vi "上传图片AOI.vi"(8 "error in (no error)":errorcluster caption="错误输入（无错误）", 10 "产品文件路径":string) -> (0 "error out":errorcluster, 1 "上传成功":bool)   [LabVIEW 2014]
uses:
  <vilib>/httpClient/MultipartData.ctl
  <vilib>/httpClient/LabVIEWHTTPClient.lvlib
panel:
  out "添加的路径":path
  out "ServerResponseBody_ANSI":string
  out "resulting string":string
  out "ServerResponseHead":string
  out "ServerResponseBody_UTF8":string
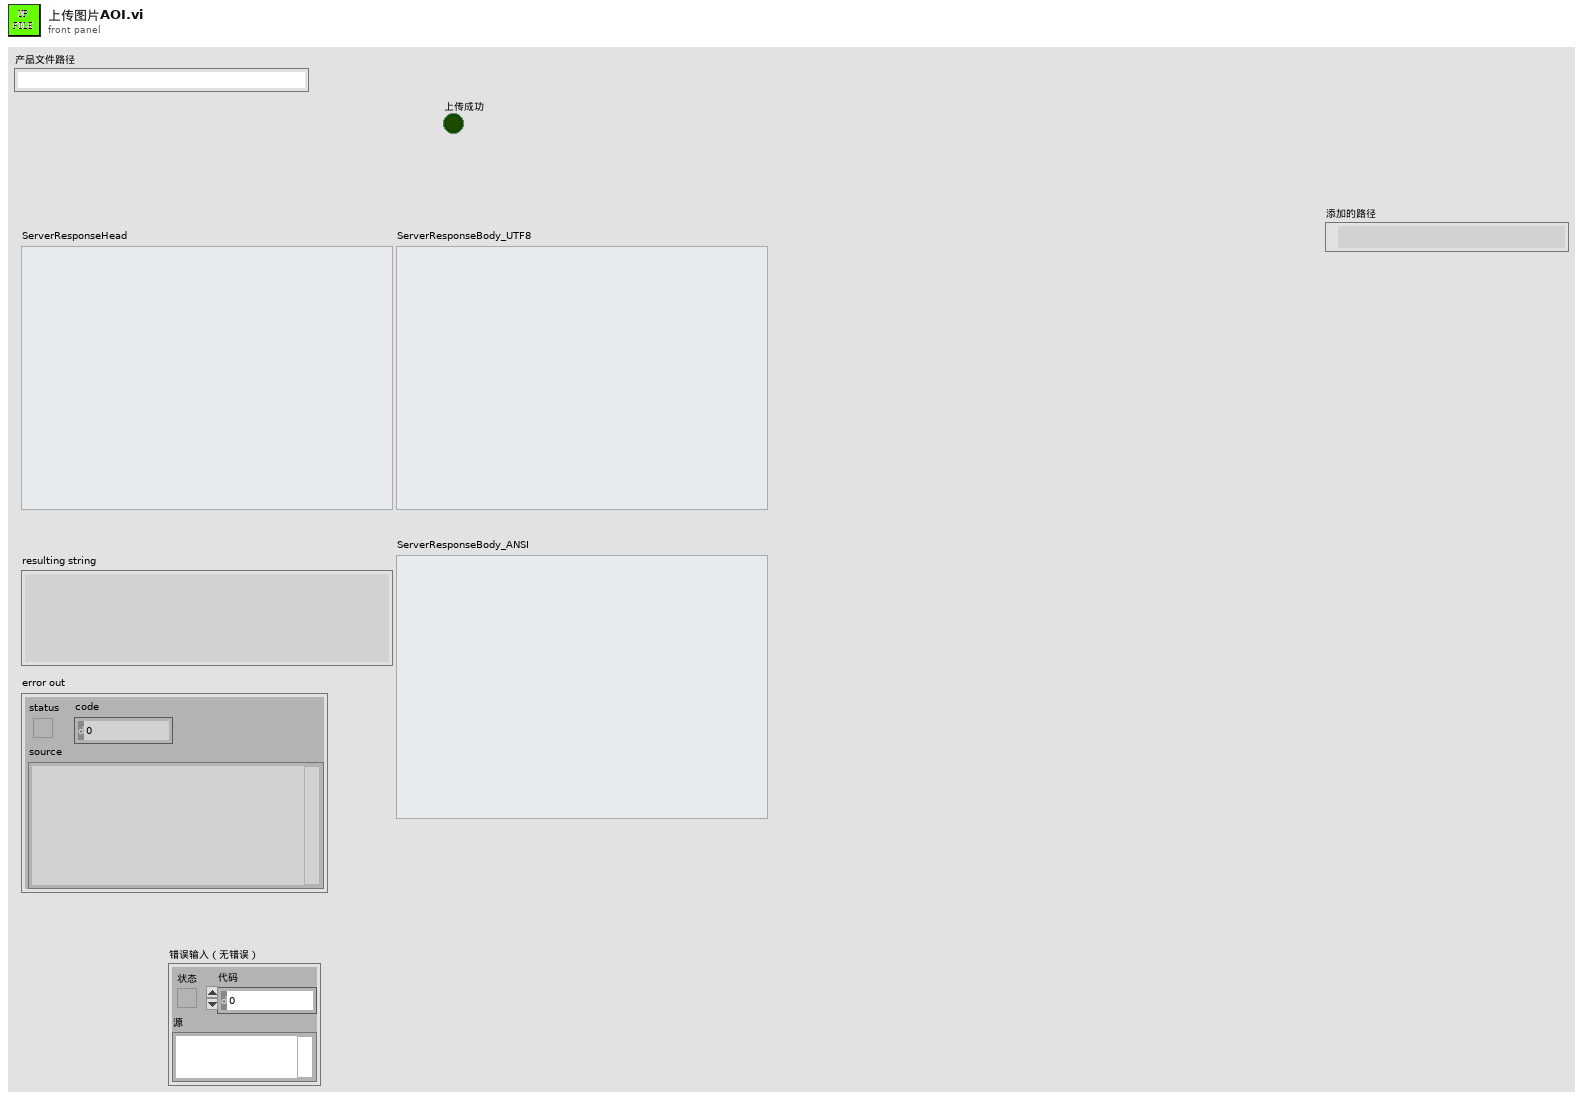
[diagram p1: front panel]
types:
  T1 = typedef "LabVIEWHTTPClient.lvlib/MultipartData.ctl" = cluster{"Name":string, "Value":string, "File":path, "Filename":string, "MIME type":string}
  T2 = typedef "LabVIEWHTTPClient.lvlib/ClientHandle.ctl" = refnum<k1>
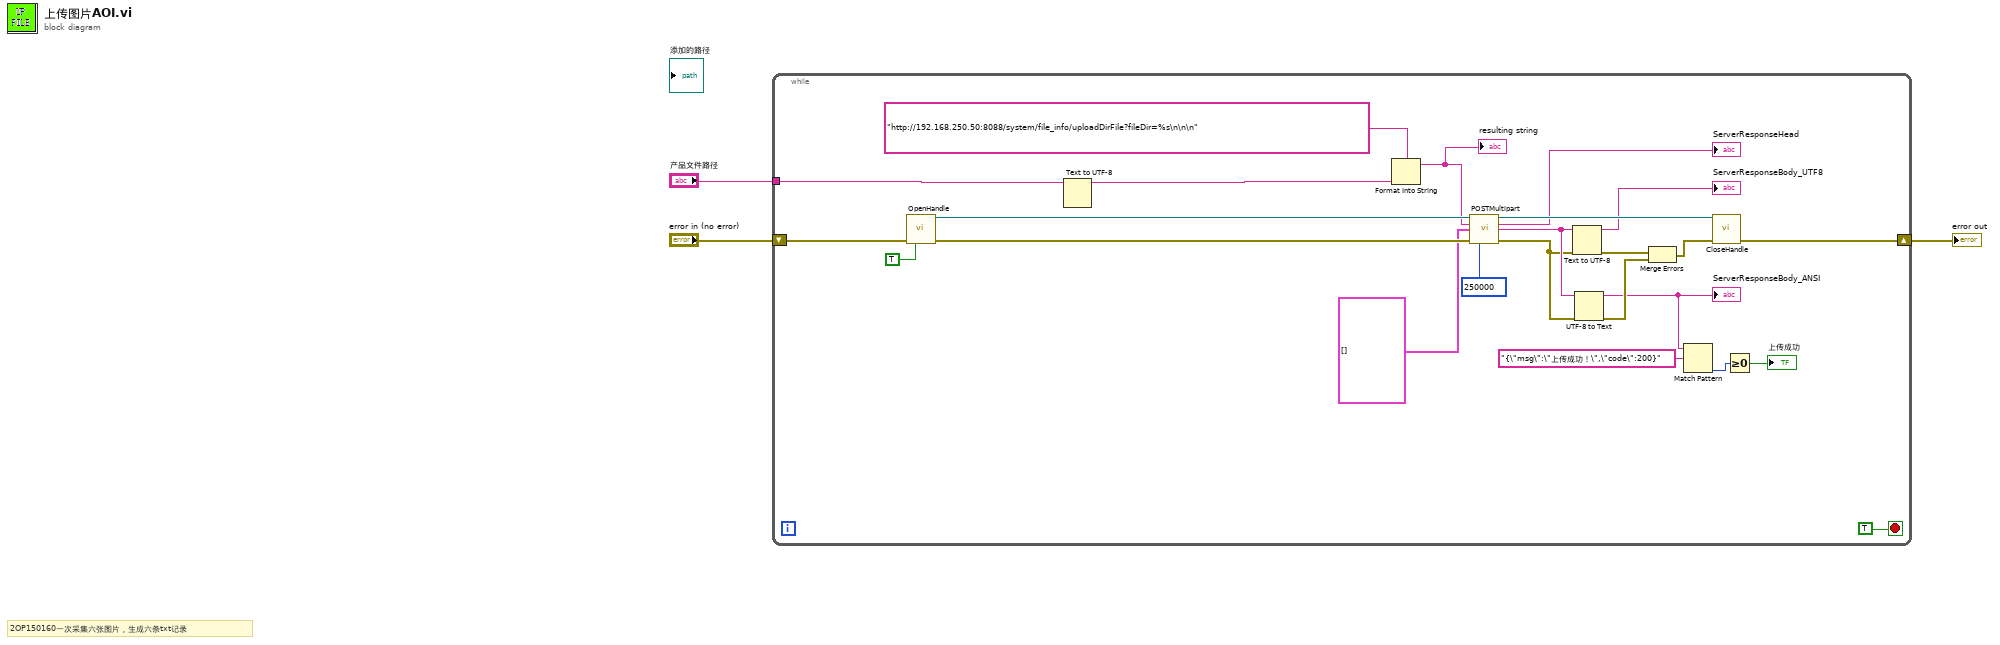
[diagram p0: block diagram]
diagram:
  # "2OP150160一次采集六张图片，生成六条txt记录"
  n1 = while {
    shift-right: [w17] -> w3
    shift-left: "error in (no error)" -> [w15]
    tunnel: "产品文件路径" -> [w10]
    stop <- TRUE stop-if-true
    n2 = call <vilib>:"OpenHandle.vi"("error in (no error)"=w15, "verify server(true)"=TRUE) -> ("client handle out"=w12:T2, "error out"=w27:errorcluster)  [unwired: 12 in]
    n3 = Text to UTF-8(11:w10) -> (3:w9:string)  [unwired: 2 in, 1 out]
    n4 = Format Into String(format string="http://192.168.250.50:8088/system/file_info/uploadDirFile?fileDir=%s\n\n\n" ("url"), w9) -> (resulting string=w8:string)  [unwired: 2 in, 1 out]
    "resulting string" <- w8
    n5 = call <vilib>:"POSTMultipart.vi"("client handle"=w12, "url"=w8, "data"=T1[] [], "error in (no error)"=w27, "timeout (10000)"=250000) -> ("client handle out"=w26:T2, "headers"=→"ServerResponseHead":string, "body"=w21:string, "error out"=w20:errorcluster)  [unwired: 7 in]
    n6 = Text to UTF-8(8:w20, 11:w21) -> (0:w19:errorcluster, 3:→"ServerResponseBody_UTF8":string)  [unwired: 1 in]
    n7 = UTF-8 to Text(8:w20, 11:w21) -> (0:w16:errorcluster, 3:w7:string)  [unwired: 1 in]
    "ServerResponseBody_ANSI" <- w7
    n8 = Merge Errors(w19, w16) -> (w18:errorcluster)
    n9 = Match Pattern(string=w7, regular expression="{\"msg\":\"上传成功！\",\"code\":200}" ("正则表达式")) -> (offset past match=w5:i32)  [unwired: 1 in, 3 out]
    n10 = call <vilib>:"CloseHandle.vi"("client handle"=w26, "error in (no error)"=w18) -> ("error out"=w17:errorcluster)  [unwired: 13 in]
    n11 = Greater Or Equal To 0?(x=w5) -> (x >= 0?=→"上传成功":bool)
  }
  "error out" <- w3
